vi "maxigauge_on_off.vi"(0 "VISA":refnum<visa-resource-name>, 1 "Channel 1":enum16{"NO CHANGE", "OFF", "ON"}(ring), 4 "Channel 2":enum16{"NO CHANGE", "OFF", "ON"}(ring), 5 "err_in":errorcluster, 10 "Channel 3":enum16{"NO CHANGE", "OFF", "ON"}(ring), 11 "Channel 4":enum16{"NO CHANGE", "OFF", "ON"}(ring), 12 "Channel 5":enum16{"NO CHANGE", "OFF", "ON"}(ring), 13 "Channel 6":enum16{"NO CHANGE", "OFF", "ON"}(ring)) -> (14 "string":string, 19 "err_out":errorcluster)   [LabVIEW 2019]
panel:
  out "status":bool
  out "status_ack":bool
  out "visa_out":refnum<visa-resource-name>
  # "Gauge status:\n1 = OFF\n2 = ON"
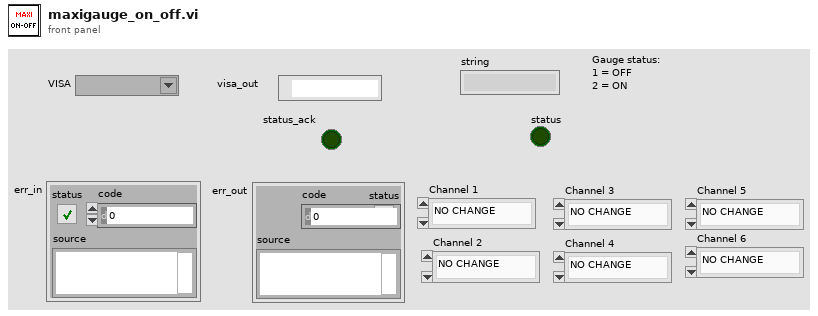
[diagram p1: front panel]
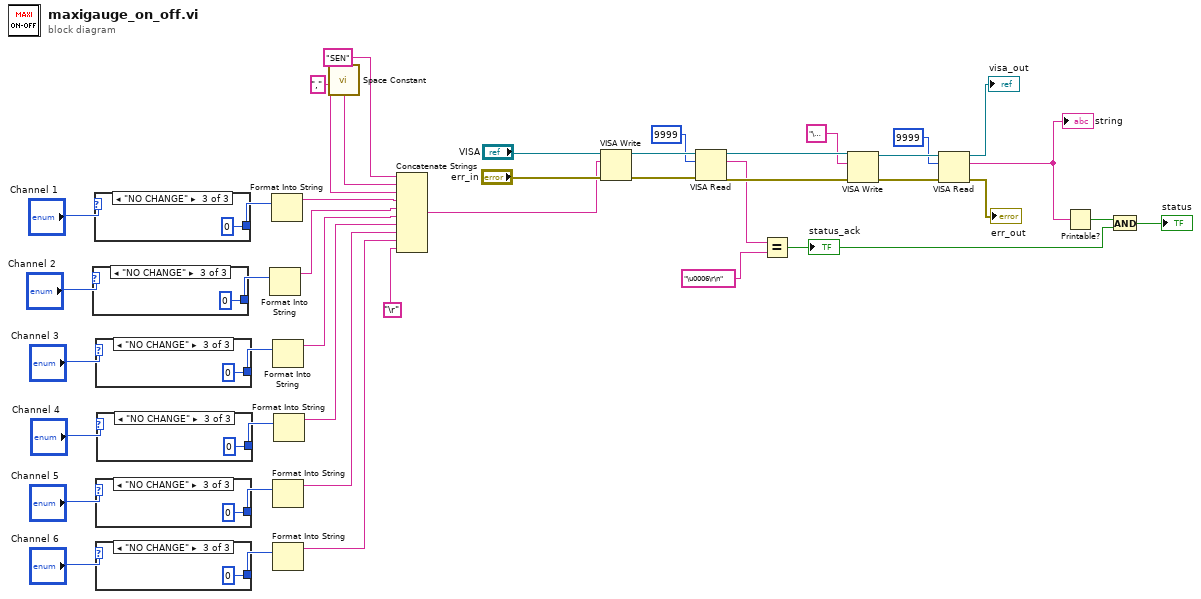
[diagram p0: block diagram]
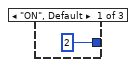
[diagram p2: hidden frame]
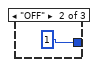
[diagram p3: hidden frame]
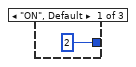
[diagram p4: hidden frame]
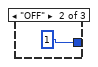
[diagram p5: hidden frame]
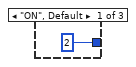
[diagram p6: hidden frame]
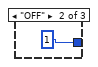
[diagram p7: hidden frame]
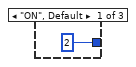
[diagram p8: hidden frame]
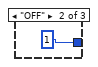
[diagram p9: hidden frame]
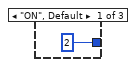
[diagram p10: hidden frame]
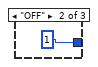
[diagram p11: hidden frame]
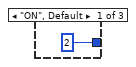
[diagram p12: hidden frame]
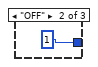
[diagram p13: hidden frame]
diagram:
  n1 = case shown="\"NO CHANGE\"" "Channel 2" {
    tunnel: [2 1 0] -> w16
    frame "ON", Default {
    }
    frame "OFF" {
    }
    frame "NO CHANGE" {
    }
  }
  n2 = case shown="\"NO CHANGE\"" "Channel 1" {
    tunnel: [2 1 0] -> w21
    frame "ON", Default {
    }
    frame "OFF" {
    }
    frame "NO CHANGE" {
    }
  }
  n3 = case shown="\"NO CHANGE\"" "Channel 3" {
    tunnel: [2 1 0] -> w13
    frame "ON", Default {
    }
    frame "OFF" {
    }
    frame "NO CHANGE" {
    }
  }
  n4 = case shown="\"NO CHANGE\"" "Channel 5" {
    tunnel: [2 1 0] -> w7
    frame "ON", Default {
    }
    frame "OFF" {
    }
    frame "NO CHANGE" {
    }
  }
  n5 = case shown="\"NO CHANGE\"" "Channel 6" {
    tunnel: [2 1 0] -> w4
    frame "ON", Default {
    }
    frame "OFF" {
    }
    frame "NO CHANGE" {
    }
  }
  n6 = case shown="\"NO CHANGE\"" "Channel 4" {
    tunnel: [2 1 0] -> w10
    frame "ON", Default {
    }
    frame "OFF" {
    }
    frame "NO CHANGE" {
    }
  }
  n7 = Format Into String(w16) -> (resulting string=w15:string)  [unwired: 3 in, 1 out]
  n8 = Format Into String(w21) -> (resulting string=w19:string)  [unwired: 3 in, 1 out]
  n9 = Format Into String(w13) -> (resulting string=w12:string)  [unwired: 3 in, 1 out]
  n10 = Format Into String(w7) -> (resulting string=w6:string)  [unwired: 3 in, 1 out]
  n11 = Format Into String(w4) -> (resulting string=w3:string)  [unwired: 3 in, 1 out]
  n12 = Format Into String(w10) -> (resulting string=w9:string)  [unwired: 3 in, 1 out]
  n13 = call <vilib>:"Space Constant.vi"() -> ("String"=w22:string)
  n14 = Concatenate Strings("SEN" ("string"), w22, "," ("string"), w19, w15, w12, w9, w6, w3, "\r") -> (w32:string)
  n15 = VISA Write(VISA resource name="VISA", write buffer=w32, error in (no error)="err_in") -> (VISA resource name out=w40:refnum<visa-resource-name>, error out=w39:errorcluster)  [unwired: 1 out]
  n16 = VISA Read(VISA resource name=w40, byte count=u32 9999, error in (no error)=w39) -> (VISA resource name out=w37:refnum<visa-resource-name>, read buffer=w30:string, error out=w38:errorcluster)  [unwired: 1 out]
  n17 = Equal?(x=w30, y="\u0006\r\n") -> (x = y?=w27:bool)
  "status_ack" <- w27
  n18 = VISA Write(VISA resource name=w37, write buffer="\u0005", error in (no error)=w38) -> (VISA resource name out=w36:refnum<visa-resource-name>, error out=w35:errorcluster)  [unwired: 1 out]
  n19 = VISA Read(VISA resource name=w36, byte count=u32 9999, error in (no error)=w35) -> (VISA resource name out=→"visa_out":refnum<visa-resource-name>, read buffer=w25:string, error out=→"err_out":errorcluster)  [unwired: 1 out]
  "string" <- w25
  n20 = Printable?(1:w25) -> (0:w24:bool)
  n21 = And(x=w24, y=w27) -> (x .and. y?=→"status":bool)
